vi "Mes Class Time.vi"(8 "error in (no error)":errorcluster, 11 "Mode":enum16{"Eight", "EModel", "Outline"}(ring)=enum."EModel") -> (0 "error out":errorcluster, 1 "结果字符串":string, 2 "Class":string, 3 "s? t:f":timestamp)   [LabVIEW 2014]
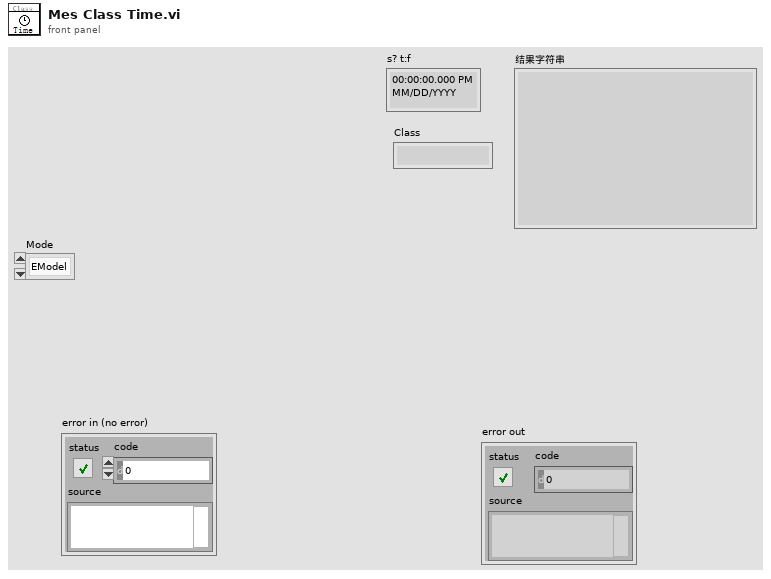
[diagram p1: front panel]
types:
  T1 = typedef "LVDateTimeRec.ctl" = cluster{"fractional second":dbl, "second":i32, "minute":i32, "hour":i32, "day of month":i32, "month":i32, "year":i32, "day of week":i32, "day of year":i32, "DST":i32}
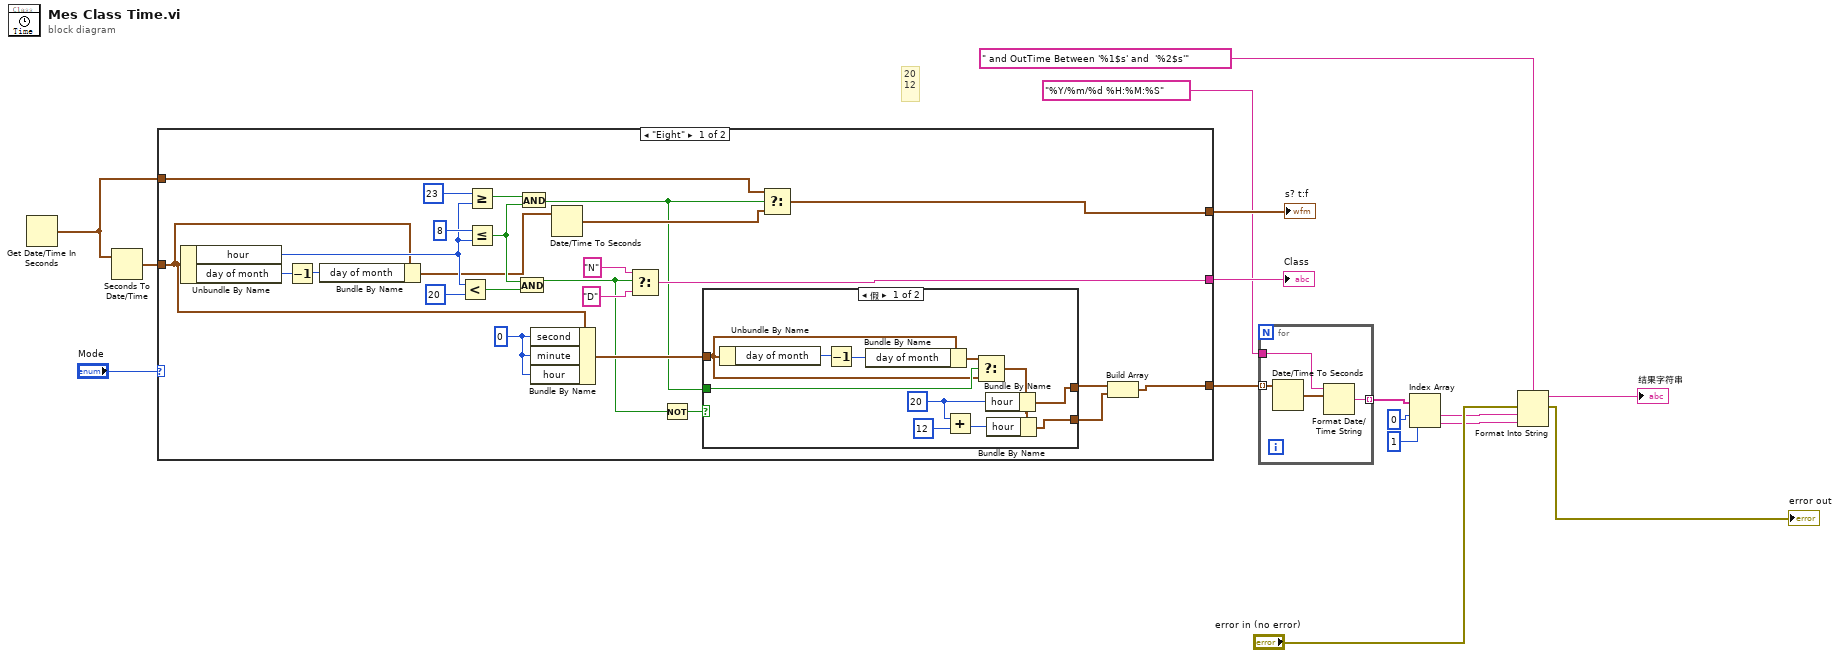
[diagram p0: block diagram]
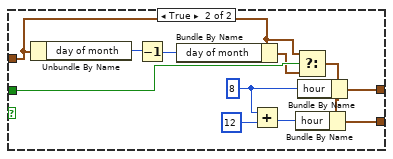
[diagram p2: hidden frame]
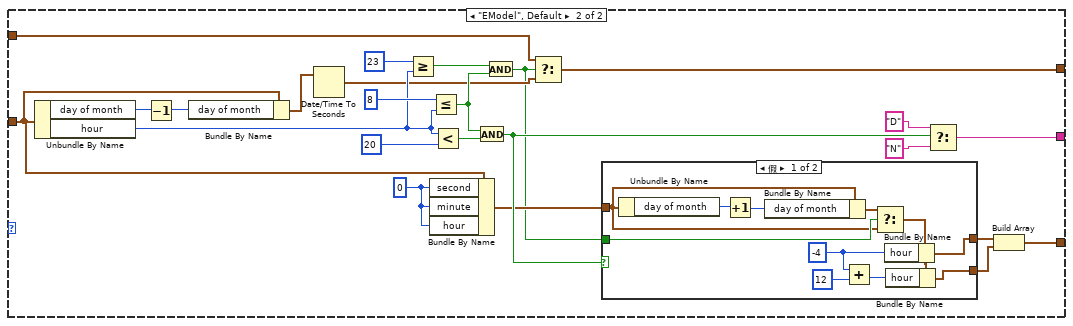
[diagram p3: hidden frame]
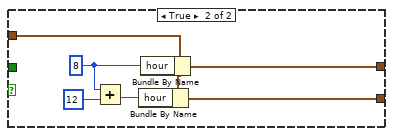
[diagram p4: hidden frame]
diagram:
  # "20\n12"
  n1 = Get Date/Time In Seconds() -> (seconds since 1Jan1904=w6:timestamp)
  n2 = Seconds To Date/Time(time stamp (now)=w6) -> (date time rec=w7:T1)  [unwired: 1 in]
  n3 = case shown="\"Eight\"" "Mode" {
    tunnel: w7 -> [w24 w70]
    tunnel: w6 -> [w31 w78]
    tunnel: [w36 w73] -> w4
    tunnel: [w26 w72] -> w5
    tunnel: [w20 w64] -> w3
    frame "Eight" {
      w25 = 0 ("second")
      n4 = Unbundle By Name(w24) -> ("hour"=w35:i32, "day of month"=w30:i32)
      n5 = Decrement(x=w30) -> (x-1=w29:i32)
      n6 = Bundle By Name(cluster=w24, "day of month"=w29) -> (w27:T1)
      n7 = Less?(x=w35, y=20) -> (x < y?=w39:bool)
      n8 = Greater Or Equal?(x=23, y=w35) -> (x >= y?=w33:bool)
      n9 = Less Or Equal?(x=8, y=w35) -> (x <= y?=w32:bool)
      n10 = And(x=w32, y=w39) -> (x .and. y?=w18:bool)
      n11 = And(x=w33, y=w32) -> (x .and. y?=w17:bool)
      n12 = Bundle By Name(cluster=w24, "second"=w25, "minute"=w25, "hour"=w25) -> (w23:T1)
      n13 = Date/Time To Seconds(2:w27) -> (0:w28:timestamp)  [unwired: 1 in]
      n14 = Select(t="N", s=w18, f="D") -> (s? t:f=w36:string)
      n15 = Not(x=w18) -> (.not. x?=w19:bool)
      n16 = case shown="假" w19 {
        tunnel: w23 -> [w48 w53]
        tunnel: w17 -> [w50 w55]
        tunnel: [w42 w60] -> w22
        tunnel: [w43 w59] -> w21
        frame False {
          w47 = 20 ("hour")
          n17 = Unbundle By Name(w48) -> ("day of month"=w52:i32)
          n18 = Decrement(x=w52) -> (x-1=w51:i32)
          n19 = Bundle By Name(cluster=w48, "day of month"=w51) -> (w49:T1)
          n20 = Add(x=w47, y=12) -> (x+y=w45:i32)
          n21 = Select(t=w49, s=w50, f=w48) -> (s? t:f=w44:T1)
          n22 = Bundle By Name(cluster=w44, "hour"=w47) -> (w42:T1)
          n23 = Bundle By Name(cluster=w44, "hour"=w45) -> (w43:T1)
        }
        frame True {
          w63 = 8 ("hour")
          n24 = Unbundle By Name(w53) -> ("day of month"=w58:i32)
          n25 = Decrement(x=w58) -> (x-1=w57:i32)
          n26 = Bundle By Name(cluster=w53, "day of month"=w57) -> (w54:T1)
          n27 = Add(x=w63, y=12) -> (x+y=w61:i32)
          n28 = Select(t=w53, s=w55, f=w54) -> (s? t:f=w56:T1)
          n29 = Bundle By Name(cluster=w56, "hour"=w61) -> (w59:T1)
          n30 = Bundle By Name(cluster=w56, "hour"=w63) -> (w60:T1)
        }
      }
      n31 = Select(t=w31, s=w17, f=w28) -> (s? t:f=w26:timestamp)
      n32 = Build Array(w22, w21) -> (w20:T1[])
    }
    frame "EModel", Default {
      w69 = 0 ("second")
      n33 = Unbundle By Name(w70) -> ("day of month"=w77:i32, "hour"=w81:i32)
      n34 = Decrement(x=w77) -> (x-1=w76:i32)
      n35 = Bundle By Name(cluster=w70, "day of month"=w76) -> (w75:T1)
      n36 = Date/Time To Seconds(2:w75) -> (0:w74:timestamp)  [unwired: 1 in]
      n37 = Greater Or Equal?(x=23, y=w81) -> (x >= y?=w79:bool)
      n38 = Bundle By Name(cluster=w70, "second"=w69, "minute"=w69, "hour"=w69) -> (w68:T1)
      n39 = Less Or Equal?(x=8, y=w81) -> (x <= y?=w80:bool)
      n40 = Less?(x=w81, y=20) -> (x < y?=w85:bool)
      n41 = And(x=w80, y=w85) -> (x .and. y?=w71:bool)
      n42 = And(x=w79, y=w80) -> (x .and. y?=w67:bool)
      n43 = Select(t=w78, s=w67, f=w74) -> (s? t:f=w72:timestamp)
      n44 = case shown="假" w71 {
        tunnel: w68 -> [w94 w101]
        tunnel: w67 -> [w96 _]
        tunnel: [w88 w100] -> w66
        tunnel: [w89 w99] -> w65
        frame False {
          w93 = -4 ("hour")
          n45 = Unbundle By Name(w94) -> ("day of month"=w98:i32)
          n46 = Increment(x=w98) -> (x+1=w97:i32)
          n47 = Bundle By Name(cluster=w94, "day of month"=w97) -> (w95:T1)
          n48 = Add(x=w93, y=12) -> (x+y=w91:i32)
          n49 = Select(t=w95, s=w96, f=w94) -> (s? t:f=w90:T1)
          n50 = Bundle By Name(cluster=w90, "hour"=w93) -> (w88:T1)
          n51 = Bundle By Name(cluster=w90, "hour"=w91) -> (w89:T1)
        }
        frame True {
          w104 = 8 ("hour")
          n52 = Add(x=w104, y=12) -> (x+y=w102:i32)
          n53 = Bundle By Name(cluster=w101, "hour"=w102) -> (w99:T1)
          n54 = Bundle By Name(cluster=w101, "hour"=w104) -> (w100:T1)
        }
      }
      n55 = Select(t="D", s=w71, f="N") -> (s? t:f=w73:string)
      n56 = Build Array(w66, w65) -> (w64:T1[])
    }
  }
  "s? t:f" <- w5
  "Class" <- w4
  n57 = for {
    tunnel: w3 -> [w108] mode=indexing
    tunnel: "%Y/%m/%d %H:%M:%S" -> [w106]
    tunnel: [w105] -> w1 mode=indexing
    n58 = Date/Time To Seconds(2:w108) -> (0:w107:timestamp)  [unwired: 1 in]
    n59 = Format Date/Time String(time format string (%c)=w106, seconds (now)=w107) -> (date/time string=w105:string)  [unwired: 1 in]
  }
  n60 = Index Array(array=w1, index #1=0 ("索引"), index #2=1 ("索引")) -> (element #1=w12:string, element #2=w11:string)
  n61 = Format Into String(format string=" and OutTime Between '%1$s' and  '%2$s'", error in="error in (no error)", w12, w11) -> (resulting string=→"结果字符串":string, error out=→"error out":errorcluster)  [unwired: 1 in]
